vi "PH_PPPA_PowerUnit.src Voltage.vi"(0 "i ref in":refnum<vi>, 2 "Voltage [V]":dbl, 5 "error in (no error)":errorcluster) -> (14 "i ref out":refnum<vi>, 19 "error out":errorcluster)   [LabVIEW 2014, in "PH_PPPA_PowerUnit.lvlib"]
doc: "This is the action VI of the Set Voltage event case. It checks whether the SM State is \"Switch PU on\" or \"Wait for Shot Cmd\" and HV off = false and Ignitron Device State = on. If this is true, it coeres the incoming voltage to the allowed range and writes it to the attributes. The voltage is written to the attributes of the SM and a state change request is send to SM for \"Set Settings\"."
uses:
  PH_PPPA_PowerUnit.lvlib
  PH_Basics/PH_StatusHandler/PH_StatusHandler.Status.ctl
  PH_Basics/PH_PowerUnit_BaseClass/PH_PowerUnit_BaseClass.SM States.ctl
  CS_Core/BaseSM/BaseSM.lvlib
  PH_Basics/PH_StatusHandler/PH_StatusHandler.lvlib
  PH_Basics/PH_Common/PH_Common.lvlib
  PH_Basics/PH_PowerUnit_BaseClass/PH_PowerUnit_BaseClass.lvlib
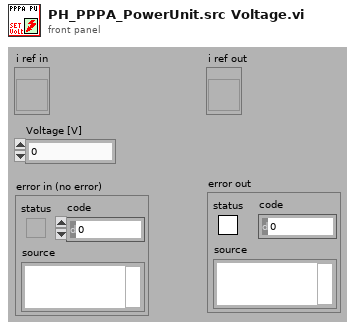
[diagram p1: front panel]
types:
  T1 = typedef "PH_PowerUnit_BaseClass.lvlib/PH_PowerUnit_BaseClass.i attribute.ctl" = cluster{"Constructor finished":bool, "PU":cluster{"In use":bool, "Service ID in use":i32, "GUI Ref":refnum<vi>}, "Enabling":cluster{"State":T2, "GUI Ref":refnum<vi>}, "Timing":cluster{"Last Shot":dbl, "Time between Shots [Sec]":dbl, "Waiting Time over?":bool, "Service ID Waiting Time":i32, "GUI Ref":refnum<vi>, "Instance":cluster{"Status":T3, "linked?":bool, "GUI Ref":refnum<vi>}}, "Sequencer":cluster{"SM State":string, "GUI Ref":refnum<vi>, "linked":bool}, "Subscribed Trendmssgs":cluster{"Tagname":string, "Status":T3, "linked?":bool, "Shot Condition":T3, "GUI Ref":refnum<vi>}[], "PP PU":T4, "Default Voltage (V)":dbl, "GUI Refs":T5, "PSDB data":cluster{"Shot Voltage [V]":dbl, "State TO SM":T6, "Write 2 early":bool}, "State TO SM":T6}
  T2 = typedef "PH_SystemInformation.lvlib/PH_SystemInformationEnabling State.ctl" = i32
  T3 = typedef "PH_StatusHandler.lvlib/PH_StatusHandler.Status.ctl" = i16
  T4 = typedef "PH_PP_Common.lvlib/PH_PP_Common.PUs.ctl" = enum16{"no Info", "PA-19mm-1", "PA-19mm-2", "PA-45mm-PILC", "PA-45mm-MAIN", "MA-PU-1", "MA-PU-2", "MA-PU-3", "MA-PU-4", "MA-PU-5", "MA-PU-6", "MA-FR", "MA-PILC", "PA-45mm-DP"}
  T5 = typedef "PH_PowerUnit_BaseClass.lvlib/PH_PowerUnit_BaseClass.GUI Refs.ctl" = cluster{"Delete Inst":refnum<vi>, "State TO SM":refnum<vi>, "State SM":refnum<vi>, "Fire":refnum<vi>}
  T6 = typedef "PH_PowerUnit_BaseClass.lvlib/PH_PowerUnit_BaseClass.SM States.ctl" = enum16{".", "Stand by", "Switch PU on", "Configure", "Set Default Voltage", "Set STANDBY", "Set READY", "Wait for Shot Cmd", "Open Dump Rods", "Open Ross Relais", "Close Ross Relais", "Switch PSU on", "Switch PSU off", "Charge", "Switch GD Channel on", "Close Dump Rods", "Rods-TO", "RR-TO", "PSU-TO", "Trigger-TO"}
  T7 = typedef "PH_PPPA_PowerUnit.lvlib/PH_PPPA_PowerUnit.i attribute.ctl" = cluster{"GUI Refs":cluster{"Ignitron":refnum<vi>, "Rossrelais":refnum<vi>, "Set Voltage":refnum<vi>, "PSU":refnum<vi>, "EOC":refnum<vi>, "Trigger":refnum<vi>}, "Ignitron":T8, "PSU":T9, "Dump Ross Relais":T10, "Trigger":cluster{"State Device":T3, "linked?":bool}, "Timing Settings":cluster{"Prdc Fast?":bool, "Default Value Periodic Interval":i32, "Mercury on since":dbl, "Warm up Time Mercury [s]":dbl}, "Set Voltage [V]":dbl, "19er Ignitionbox":string}
  T8 = typedef "PH_PP_Common.lvlib/PH_PP_Common.Ignitron Attributes.ctl" = cluster{"State Device":T3, "linked?":bool}
  T9 = typedef "PH_PP_Common.lvlib/PH_PP_Common.PSU Attributes.ctl" = cluster{"lower limit [V]":dbl, "upper limit [V]":dbl, "Voltage set":bool, "State Device":T3, "linked?":bool}
  T10 = typedef "PH_PP_Common.lvlib/PH_PP_Common.Ross Relais Attributes.ctl" = cluster{"State Device":T3, "linked?":bool}
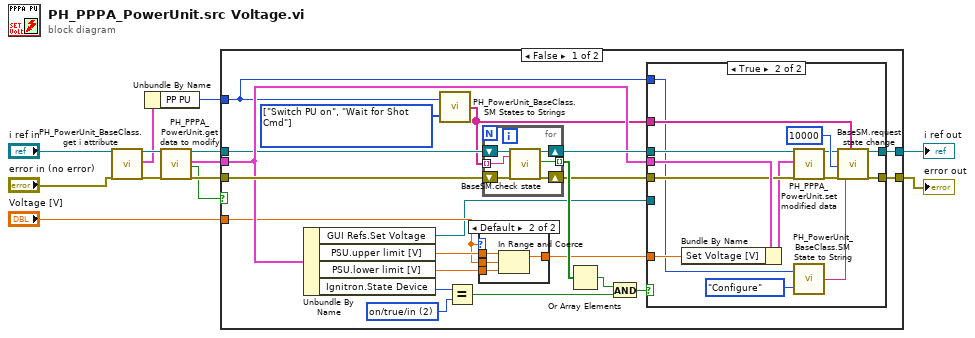
[diagram p0: block diagram]
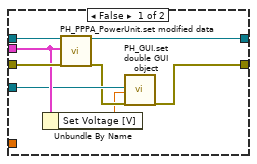
[diagram p3: hidden frame]
diagram:
  n1 = call "PH_PowerUnit_BaseClass.get i attribute.vi"("i ref in"="i ref in", "error in (no error)"="error in (no error)") -> ("i ref out"=w3:refnum<vi>, "i attribute"=w2:T1, "error out"=w5:errorcluster)  [unwired: 15 in]
  n2 = Unbundle By Name(w2) -> ("PP PU"=w1:T4)
  n3 = call "PH_PPPA_PowerUnit.get data to modify.vi"("i ref in"=w3, "error in (no error)"=w5) -> ("i ref out"=w10:refnum<vi>, "i attribute"=w13:T7, "timed out"=w7:bool, "error out"=w11:errorcluster)  [unwired: 14 in]
  n4 = case shown="False" w7 {
    tunnel: w13 -> [w25 _]
    tunnel: w11 -> [w32 w68]
    tunnel: w10 -> [w20 w69]
    tunnel: [w18 w69] -> w9
    tunnel: [w19 w68] -> w8
    tunnel: "Voltage [V]" -> [w24 _]
    tunnel: w1 -> [w14 _]
    frame False {
      w16 = T6[] [enum."Switch PU on", enum."Wait for Shot Cmd"] items=[".", "Stand by", "Switch PU on", "Configure", "Set Default Voltage", "Set STANDBY", "Set READY", "Wait for Shot Cmd", "Open Dump Rods", "Open Ross Relais", "Close Ross Relais", "Switch PSU on", "Switch PSU off", "Charge", "Switch GD Channel on", "Close Dump Rods", "Rods-TO", "RR-TO", "PSU-TO", "Trigger-TO"] ("SM States")
      w17 = T3 2 items=["no info", "off/false/out", "on/true/in", "Failure", "Alarm", "Status 1", "Status 2", "Status 3"] ("Ignitron.State Device")
      n5 = Unbundle By Name(w25) -> ("GUI Refs.Set Voltage"=w22:refnum<vi>, "PSU.upper limit [V]"=w26:dbl, "PSU.lower limit [V]"=w27:dbl, "Ignitron.State Device"=w30:T3)
      n6 = call "PH_PowerUnit_BaseClass.SM States to Strings.vi"("SM States"=w16, "PU"=w14) -> ("SM State Strings"=w15:string[])
      n7 = Equal?(x=w30, y=w17) -> (x = y?=w29:bool)
      n8 = case shown="Default" w24 {
        tunnel: w27 -> [_ w39]
        tunnel: w26 -> [_ w38]
        tunnel: w24 -> [w35 w37]
        tunnel: [w35 w36] -> w23
        frame 0 {
        }
        frame Default {
          n9 = In Range and Coerce(upper limit=w38, x=w37, lower limit=w39) -> (coerced(x)=w36:dbl)  [unwired: 1 out]
        }
      }
      n10 = for {
        shift-right: [w44] -> w31
        shift-left: w32 -> [w45]
        shift-right: [w43] -> w33
        shift-left: w20 -> [w42]
        tunnel: w15 -> [w41] mode=indexing
        tunnel: [w40] -> w34 mode=indexing
        n11 = call "BaseSM.check state.vi"("i ref in"=w42, "requestedState"=w41, "error in (no error)"=w45) -> ("i ref out"=w43:refnum<vi>, "OK"=w40:bool, "error out"=w44:errorcluster)  [unwired: 11 in, 3 out]
      }
      n12 = Or Array Elements(Boolean array=w34) -> (logical OR=w28:bool)
      n13 = And(x=w28, y=w29) -> (x .and. y?=w21:bool)
      n14 = case shown="True" w21 {
        tunnel: [w47 w67] -> w19
        tunnel: w33 -> [w53 w61]
        tunnel: w31 -> [w51 w59]
        tunnel: w15 -> [_ w66]
        tunnel: w25 -> [w50 w65]
        tunnel: w23 -> [_ w64]
        tunnel: w22 -> [w49 _]
        tunnel: [w52 w62] -> w18
        tunnel: w14 -> [_ w54]
        frame False {
          n15 = Unbundle By Name(w50) -> ("Set Voltage [V]"=w46:dbl)
          n16 = call "PH_PPPA_PowerUnit.set modified data.vi"("i ref in"=w53, "i attribute"=w50, "error in (no error)"=w51) -> ("i ref out"=w52:refnum<vi>, "error out"=w48:errorcluster)  [unwired: 15 in]
          n17 = call "PH_GUI.set double GUI object.vi"("GUI object Ref"=w49, "value"=w46, "error in (no error)"=w48) -> ("error out"=w47:errorcluster)  [unwired: 16 in]
        }
        frame True {
          n18 = Bundle By Name(cluster=w65, "Set Voltage [V]"=w64) -> (w57:T7)
          n19 = call "PH_PPPA_PowerUnit.set modified data.vi"("i ref in"=w61, "i attribute"=w57, "error in (no error)"=w59) -> ("i ref out"=w60:refnum<vi>, "error out"=w58:errorcluster)  [unwired: 15 in]
          n20 = call "PH_PowerUnit_BaseClass.SM State to String.vi"("SM State"=PH_PowerUnit_BaseClass.SM_States."Configure", "PU"=w54) -> ("SM State String"=w56:string)
          n21 = call "BaseSM.request state change.vi"("i ref in"=w60, "ms timeout (10000)"=10000 ("ms timeout (-1)"), "error in (no error)"=w58, "requested state"=w56, "allowed current states"=w66) -> ("i ref out"=w62:refnum<vi>, "error out"=w67:errorcluster)  [unwired: 11 in, 2 out]
        }
      }
    }
    frame True {
    }
  }
  "i ref out" <- w9
  "error out" <- w8
